vi "Transition Measurements 1 chan (old method).vi"(6 "percent level settings":T3={"method"=enum."auto select", "histogram size"=256, "histogram method"=enum."mode", "reserved"=1.0} {"reserved" format="%0.2f"}, 7 "edge number (1)":i32=1 min=1, 8 "error in (no error)":errorcluster, 9 "reference levels":T4={"high ref level"=90.0, "mid ref level"=50.0, "low ref level"=10.0, "ref units"=1} {"ref units" items=["absolute", "percent"]; "high ref level" format="%0.2f"; "low ref level" format="%0.2f"; "mid ref level" format="%0.2f"}, 10 "polarity (rising)":u16(ring)=1 items=["falling", "rising"], 11 "signal in":waveform(dbl)={"t0"=timestamp(0 s since 1904-01-01), "dt"=0.0, "Y"=[]}) -> (0 "error out":errorcluster, 1 "post-transition":T1, 2 "pre-transition":T1, 3 "transition duration":dbl, 4 "measurement info":T2 {"ref levels"."ref units" items=["absolute", "relative"]; "ref levels"."high ref level" format="%.2p"; "ref levels"."low ref level" format="%.2p"; "ref levels"."mid ref level" format="%.2p"; "end time" format="%.2p"; "start time" format="%.2p"}, 5 "slope":dbl)   [LabVIEW 2020, in "NI_MAPro.lvlib"]
uses:
  NI_MAPro.lvlib
  <resource>/lvanlys.dll
  NI_MABase.lvlib
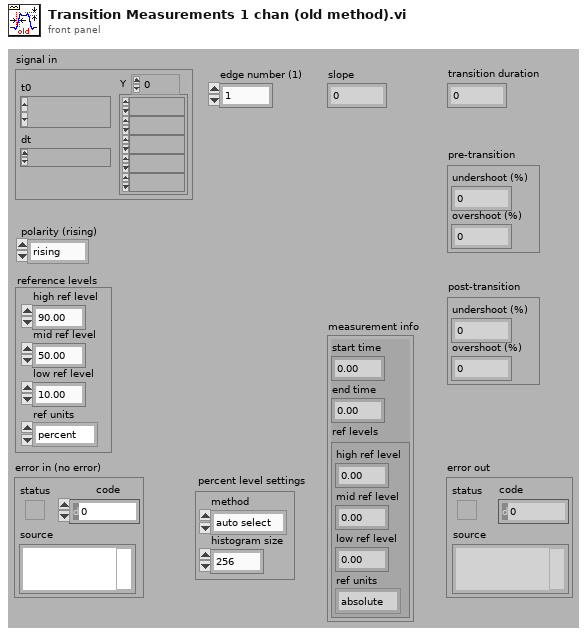
[diagram p1: front panel]
types:
  T1 = cluster{"undershoot (%)":dbl, "overshoot (%)":dbl}
  T2 = cluster{"start time":dbl, "end time":dbl, "ref levels":cluster{"high ref level":dbl, "mid ref level":dbl, "low ref level":dbl, "ref units":u16}}
  T3 = cluster{"method":enum32{"histogram", "peak", "auto select"}, "histogram size":i32, "histogram method":enum16{"mode"}, "reserved":dbl}
  T4 = cluster{"high ref level":dbl, "mid ref level":dbl, "low ref level":dbl, "ref units":u16}
  T5 = cluster{"PostUnderShoot":dbl, "PostOverShoot":dbl}
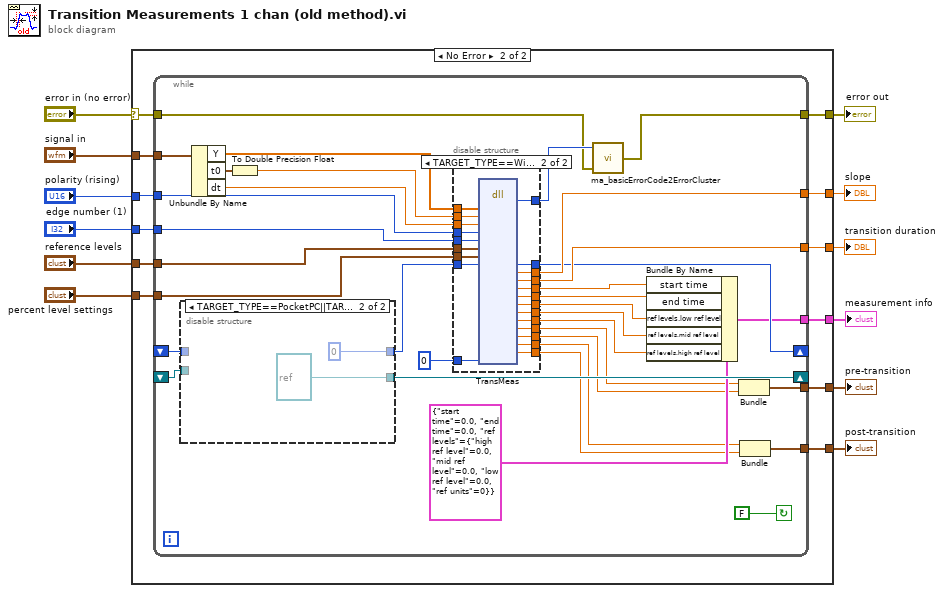
[diagram p0: block diagram]
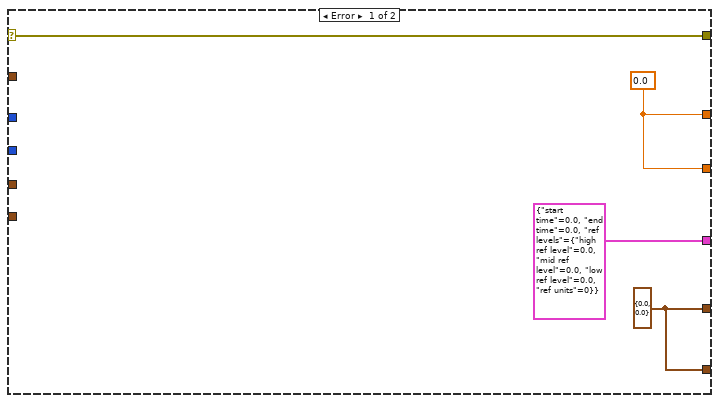
[diagram p2: hidden frame]
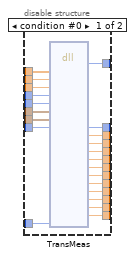
[diagram p3: hidden frame]
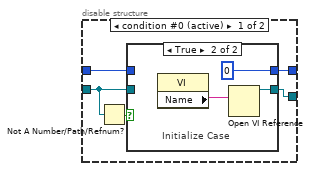
[diagram p4: hidden frame]
diagram:
  n1 = case shown="No Error" "error in (no error)" {
    selector: "error in (no error)" -> [w16 w27]
    tunnel: "polarity (rising)" -> [_ w22]
    tunnel: "reference levels" -> [_ w24]
    tunnel: "percent level settings" -> [_ w25]
    tunnel: "edge number (1)" -> [_ w23]
    tunnel: "signal in" -> [_ w28]
    tunnel: [T2 {"start time"=0.0, "end time"=0.0, "ref levels"={"high ref level"=0.0, "mid ref level"=0.0, "low ref level"=0.0, "ref units"=0}} ("measurement info") w19] -> w3
    tunnel: [w16 w26] -> w6
    tunnel: [w15 w20] -> w5
    tunnel: [w15 w21] -> w4
    tunnel: [w13 w18] -> w2
    tunnel: [w13 w17] -> w1
    frame Error {
      w13 = cluster{"PreUnderShoot":dbl, "PreOverShoot":dbl} {"PreUnderShoot"=0.0, "PreOverShoot"=0.0}
      w15 = 0.0 ("result")
    }
    frame No Error {
      n2 = while {
        tunnel: w28 -> [w62]
        tunnel: w27 -> [w30]
        tunnel: [w29] -> w26
        tunnel: [w40] -> w19
        tunnel: w25 -> [w60]
        tunnel: w24 -> [w59]
        tunnel: w23 -> [w58]
        tunnel: w22 -> [w57]
        tunnel: [w52] -> w21
        tunnel: [w51] -> w20
        shift-right: [w50] -> _
        shift-left: _ -> [w44]
        shift-right: [w41] -> _
        shift-left: _ -> [w43]
        tunnel: [w36] -> w18
        tunnel: [w33] -> w17
        stop <- FALSE continue-if-true
        n3 = disable-structure shown="TARGET_TYPE==PocketPC||TARGET_TYPE==PalmOS||TARGET_TYPE==FPGA||TARGET_TYPE==Embedded" {
          disable-tunnel: w43 -> [w109 _]
          disable-tunnel: [w110 refnum<vi> refnum ("VI Refnum")] -> w41
          disable-tunnel: w44 -> [w108 _]
          disable-tunnel: [w107 0 ("t")] -> w42
          frame condition #0 (active) {
            n4 = Not A Number/Path/Refnum?(number/path/refnum=w109) -> (NaN/Path/Refnum?=w111:bool)
            n5 = case shown="True" w111 {
              tunnel: [w113 w115] -> w110
              tunnel: w109 -> [w113 _]
              tunnel: w108 -> [w112 _]
              tunnel: [w112 0 ("error")] -> w107
              frame False {
              }
              frame True {
                # "Initialize Case"
                n6 = property class="VI"() -> ("Name"=w114:string)  [unwired: 2 in, 2 out]
                n7 = Open VI Reference(vi path=w114) -> (vi reference=w115:refnum<vi>)  [unwired: 1 in, 5 out]
              }
            }
          }
          frame condition #1 {
          }
        }
        n8 = Unbundle By Name(w62) -> ("Y"=w61:dbl[], "t0"=w56:timestamp, "dt"=w54:dbl)
        n9 = To Double Precision Float(number=w56) -> (double precision float=w55:dbl)
        n10 = disable-structure shown="TARGET_TYPE==Windows||TARGET_TYPE==Mac||TARGET_TYPE==Unix||TARGET_BITNESS==64" {
          disable-tunnel: w61 -> [w84 w106]
          disable-tunnel: [w83 w105] -> w31
          disable-tunnel: w60 -> [w82 w104]
          disable-tunnel: w59 -> [w81 w103]
          disable-tunnel: w58 -> [w80 w102]
          disable-tunnel: w57 -> [w79 w101]
          disable-tunnel: w55 -> [w78 w100]
          disable-tunnel: w54 -> [w77 w99]
          disable-tunnel: [w76 w98] -> w52
          disable-tunnel: [w75 w97] -> w51
          disable-tunnel: [w74 w96] -> w50
          disable-tunnel: [w73 w95] -> w49
          disable-tunnel: [w72 w94] -> w48
          disable-tunnel: [w71 w93] -> w47
          disable-tunnel: [w70 w92] -> w46
          disable-tunnel: [w69 w91] -> w45
          disable-tunnel: w42 -> [w68 w90]
          disable-tunnel: [w67 w89] -> w38
          disable-tunnel: [w66 w88] -> w37
          disable-tunnel: [w65 w87] -> w35
          disable-tunnel: [w64 w86] -> w34
          disable-tunnel: 0 ("newAlgorithm") -> [w63 w85]
          frame condition #0 {
            n11 = dll-call lib="C:/Program Files (x86)/National Instruments/LabVIEW 2020/resource/lvanlys.*" fn="TransMeas"("xH"=w84, "Xo"=w78, "dx"=w77, "polarity"=w79, "edgeNum"=w80, "refLevel"=w81, "percentLevel"=w82, "work"=w68, "newAlgorithm"=w63) -> ("return type"=w83:i32, "work"=w74:i32, "slewRate"=w75:dbl, "transDuration"=w76:dbl, "startingTime"=w73:dbl, "endingTime"=w72:dbl, "lowRefLevel"=w71:dbl, "midRefLevel"=w70:dbl, "highRefLevel"=w69:dbl, "PreUnderShoot"=w67:dbl, "PreOverShoot"=w66:dbl, "PostUnderShoot"=w65:dbl, "PostOverShoot"=w64:dbl)  [unwired: 22 in, 2 out]
          }
          frame condition #1 (active) {
            n12 = dll-call lib="C:/Program Files (x86)/National Instruments/LabVIEW 2020/resource/lvanlys.dll" fn="TransMeas"("xH"=w106, "Xo"=w100, "dx"=w99, "polarity"=w101, "edgeNum"=w102, "refLevel"=w103, "percentLevel"=w104, "work"=w90, "newAlgorithm"=w85) -> ("return type"=w105:i32, "work"=w96:i64, "slewRate"=w97:dbl, "transDuration"=w98:dbl, "startingTime"=w95:dbl, "endingTime"=w94:dbl, "lowRefLevel"=w93:dbl, "midRefLevel"=w92:dbl, "highRefLevel"=w91:dbl, "PreUnderShoot"=w89:dbl, "PreOverShoot"=w88:dbl, "PostUnderShoot"=w87:dbl, "PostOverShoot"=w86:dbl)  [unwired: 9 in, 15 out]
          }
        }
        n13 = call "ma_basicErrorCode2ErrorCluster.vi"("error in (no error)"=w30, "Error Code"=w31) -> ("error out"=w29:errorcluster)  [unwired: 1 in]
        n14 = Bundle By Name(cluster=T2 {"start time"=0.0, "end time"=0.0, "ref levels"={"high ref level"=0.0, "mid ref level"=0.0, "low ref level"=0.0, "ref units"=0}} ("measurement info"), "start time"=w49, "end time"=w48, "ref levels.low ref level"=w47, "ref levels.mid ref level"=w46, "ref levels.high ref level"=w45) -> (w40:T2)
        n15 = Bundle("PreUnderShoot"=w38, "PreOverShoot"=w37) -> (w36:cluster{"PreUnderShoot":dbl, "PreOverShoot":dbl})  [unwired: 1 out]
        n16 = Bundle("PostUnderShoot"=w35, "PostOverShoot"=w34) -> (w33:T5)  [unwired: 1 out]
      }
    }
  }
  "slope" <- w5
  "transition duration" <- w4
  "measurement info" <- w3
  "error out" <- w6
  "post-transition" <- w1
  "pre-transition" <- w2
